vi "FTP upload HTML map.vi"(11 "Name of Exchange":string) -> ()   [LabVIEW 2010]
panel:
  out "standard output":string
  out "error out":errorcluster
  out "standard error":string
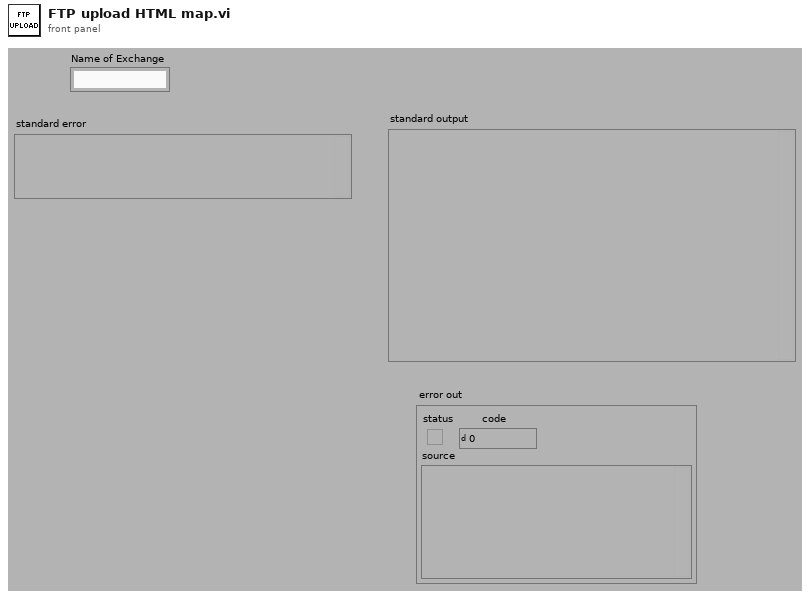
[diagram p1: front panel]
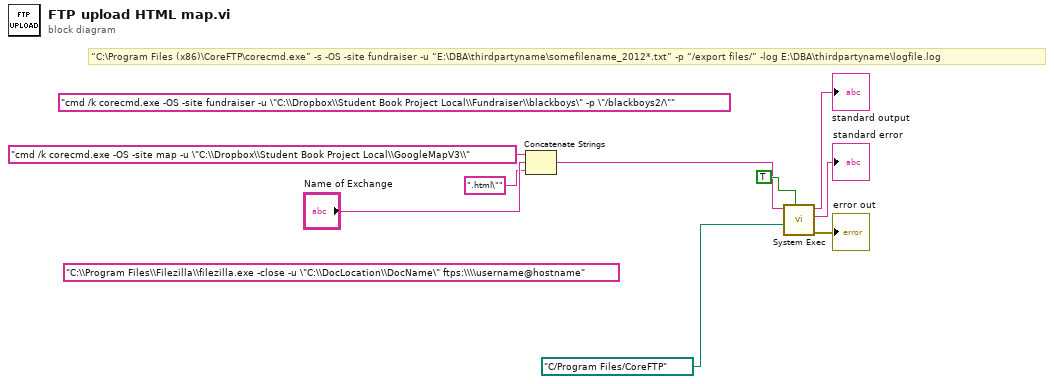
[diagram p0: block diagram]
diagram:
  (unwired) "C:\\Program Files\\Filezilla\\filezilla.exe -close -u \"C:\\DocLocation\\DocName\" ftps:\\\\username@hostname"
  (unwired) "cmd /k corecmd.exe -OS -site fundraiser -u \"C:\\Dropbox\\Student Book Project Local\\Fundraiser\\blackboys\" -p \"/blackboys2/\"" ("command line")
  # "“C:\\Program Files (x86)\\CoreFTP\\corecmd.exe” -s -OS -site fundraiser -u “E:\\DBA\\thirdpartyname\\somefilename_2012*.txt” -p “/export files/” -log E:\\DBA\\thirdpartyname\\logfile.log"
  n1 = Concatenate Strings("cmd /k corecmd.exe -OS -site map -u \"C:\\Dropbox\\Student Book Project Local\\GoogleMapV3\\" ("string"), "Name of Exchange", ".html\"" ("string")) -> (w1:string)
  n2 = call <vilib>:"System Exec.vi"("wait until completion? (T)"=TRUE, "working directory"=path "C:/Program Files/CoreFTP", "command line"=w1) -> ("error out"=→"error out":errorcluster, "standard error"=→"standard error":string, "standard output"=→"standard output":string)  [unwired: 5 in, 1 out]
